vi "Generate Service Config JSON.vi"(0 "service descriptor":T3, 5 "provided interfaces":string[](array[string]), 7 "path":string, 11 "error in":errorcluster) -> (4 "service config JSON":string, 15 "error out":errorcluster)   [LabVIEW 2021, in "NI Measurement Plug-In SDK.lvlib"]
uses:
  NI Measurement Plug-In SDK.lvlib
  TypeDefs/Measurement Details.ctl
  TypeDefs/Measurement Annotation.ctl
  867c5996-9fc4-446f-bc7e-cd1af3184270.vi
  3e130467-15fc-4370-9f76-fa76b7d976c8.vi
  a066e80c-61f1-4c64-8e78-6e3d97fd6b7b.vi
  2858ca83-f95f-4d85-8bb1-5ba8a53c7693.vi
  26abaa1b-7193-4077-a3e4-3b2bfa2f984b.vi
  b2866af8-bc70-4c0d-b595-9f5224cfa858.vi
  0c37daab-07df-4eb5-bca5-1a967d50c5e0.vi
  867c5996-9fc4-446f-bc7e-cd1af3184270.vi/49d2641b-58d2-418d-86ef-5c98235809e6.vi
  867c5996-9fc4-446f-bc7e-cd1af3184270.vi/729eb87d-9ab4-481c-bd0a-7090d6acb718.vi
  3e130467-15fc-4370-9f76-fa76b7d976c8.vi/49d2641b-58d2-418d-86ef-5c98235809e6.vi
  3e130467-15fc-4370-9f76-fa76b7d976c8.vi/729eb87d-9ab4-481c-bd0a-7090d6acb718.vi
  a066e80c-61f1-4c64-8e78-6e3d97fd6b7b.vi/49d2641b-58d2-418d-86ef-5c98235809e6.vi
  a066e80c-61f1-4c64-8e78-6e3d97fd6b7b.vi/729eb87d-9ab4-481c-bd0a-7090d6acb718.vi
  2858ca83-f95f-4d85-8bb1-5ba8a53c7693.vi/49d2641b-58d2-418d-86ef-5c98235809e6.vi
  2858ca83-f95f-4d85-8bb1-5ba8a53c7693.vi/729eb87d-9ab4-481c-bd0a-7090d6acb718.vi
  26abaa1b-7193-4077-a3e4-3b2bfa2f984b.vi/49d2641b-58d2-418d-86ef-5c98235809e6.vi
  26abaa1b-7193-4077-a3e4-3b2bfa2f984b.vi/729eb87d-9ab4-481c-bd0a-7090d6acb718.vi
  b2866af8-bc70-4c0d-b595-9f5224cfa858.vi/49d2641b-58d2-418d-86ef-5c98235809e6.vi
  b2866af8-bc70-4c0d-b595-9f5224cfa858.vi/729eb87d-9ab4-481c-bd0a-7090d6acb718.vi
  0c37daab-07df-4eb5-bca5-1a967d50c5e0.vi/49d2641b-58d2-418d-86ef-5c98235809e6.vi
  0c37daab-07df-4eb5-bca5-1a967d50c5e0.vi/729eb87d-9ab4-481c-bd0a-7090d6acb718.vi
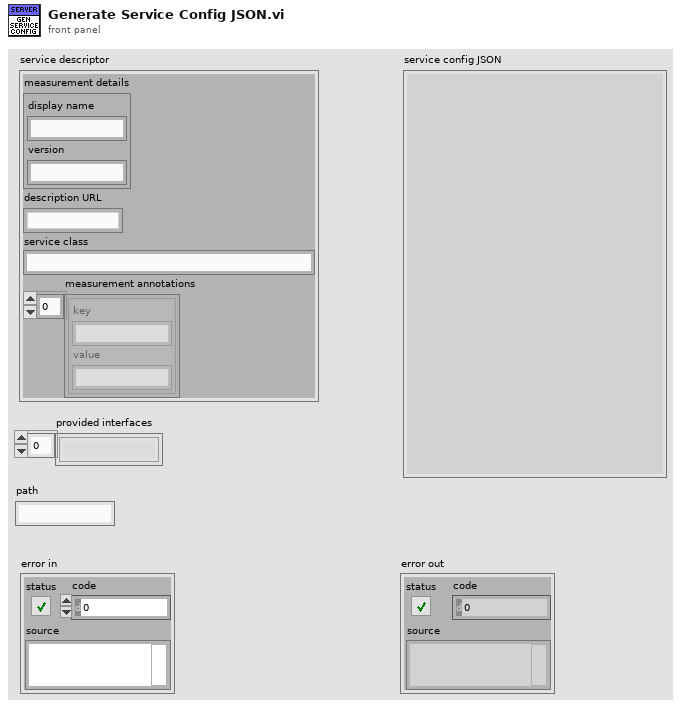
[diagram p1: front panel]
types:
  T1 = typedef "NI Measurement Plug-In SDK.lvlib/Measurement Details.ctl" = cluster{"display name":string, "version":string}
  T2 = typedef "NI Measurement Plug-In SDK.lvlib/Measurement Annotation.ctl" = cluster{"key":string, "value":string}
  T3 = cluster{"measurement details":T1, "description URL":string, "service class":string, "measurement annotations":T2[]}
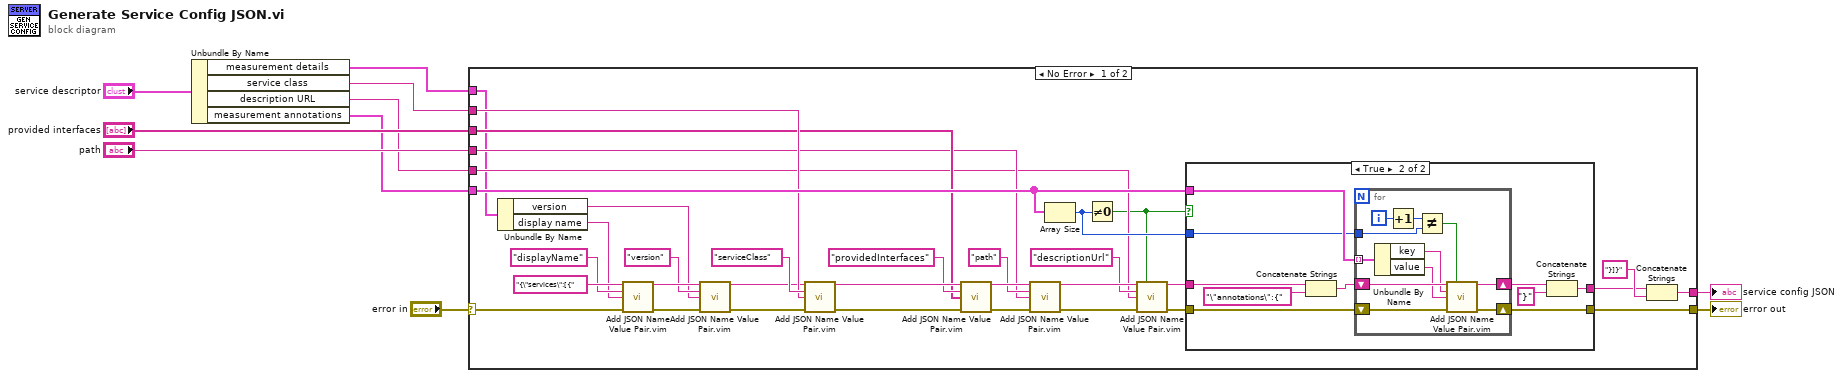
[diagram p0: block diagram]
diagram:
  n1 = Unbundle By Name("service descriptor") -> ("measurement details"=w4:T1, "service class"=w3:string, "description URL"=w2:string, "measurement annotations"=w1:T2[])
  n2 = case shown="No Error" "error in" {
    selector: "error in" -> [w38 w68]
    tunnel: [w42 w68] -> w9
    tunnel: w4 -> [w16 _]
    tunnel: w3 -> [w34 _]
    tunnel: "provided interfaces" -> [w30 _]
    tunnel: [w43 _] -> w7
    tunnel: "path" -> [w26 _]
    tunnel: w2 -> [w21 _]
    tunnel: w1 -> [w41 _]
    frame No Error {
      n3 = Unbundle By Name(w16) -> ("version"=w12:string, "display name"=w15:string)
      n4 = call "Add JSON Name Value Pair.vim"("JSON string in"="{\"services\":[{", "name"="displayName", "value"=w15, "error in"=w38) -> ("JSON string out"=w14:string, "error out"=w18:errorcluster)  [unwired: 10 in]
      n5 = call "Add JSON Name Value Pair.vim"("JSON string in"=w14, "name"="version", "value"=w12, "error in"=w18) -> ("JSON string out"=w11:string, "error out"=w17:errorcluster)  [unwired: 10 in]
      n6 = call "Add JSON Name Value Pair.vim"("JSON string in"=w11, "name"="serviceClass", "value"=w34, "error in"=w17) -> ("JSON string out"=w32:string, "error out"=w33:errorcluster)  [unwired: 10 in]
      n7 = call "Add JSON Name Value Pair.vim"("JSON string in"=w32, "name"="providedInterfaces", "value"=w30, "error in"=w33) -> ("JSON string out"=w28:string, "error out"=w29:errorcluster)  [unwired: 10 in]
      n8 = call "Add JSON Name Value Pair.vim"("JSON string in"=w28, "name"="path", "value"=w26, "error in"=w29) -> ("JSON string out"=w23:string, "error out"=w25:errorcluster)  [unwired: 10 in]
      n9 = Array Size(array=w41) -> (size(s)=w40:i32)
      n10 = Not Equal To 0?(x=w40) -> (x != 0?=w20:bool)
      n11 = call "Add JSON Name Value Pair.vim"("JSON string in"=w23, "include trailing comma"=w20, "name"="descriptionUrl", "value"=w21, "error in"=w25) -> ("JSON string out"=w19:string, "error out"=w24:errorcluster)  [unwired: 9 in]
      n12 = case shown="True" w20 {
        tunnel: w24 -> [w46 w56]
        tunnel: [w46 w55] -> w42
        tunnel: w41 -> [_ w54]
        tunnel: w40 -> [_ w51]
        tunnel: [w45 w48] -> w39
        tunnel: w19 -> [w45 w47]
        frame False {
        }
        frame True {
          n13 = Concatenate Strings(w47, "\"annotations\":{") -> (w52:string)
          n14 = for {
            shift-right: [w62] -> w55
            shift-left: w56 -> [w63]
            tunnel: w54 -> [w65] mode=indexing
            shift-right: [w60] -> w50
            shift-left: w52 -> [w61]
            tunnel: w51 -> [w64]
            i -> [w67]
            n15 = Unbundle By Name(w65) -> ("key"=w57:string, "value"=w58:string)
            n16 = Increment(x=w67) -> (x+1=w66:i32)
            n17 = Not Equal?(x=w66, y=w64) -> (x != y?=w59:bool)
            n18 = call "Add JSON Name Value Pair.vim"("JSON string in"=w61, "include trailing comma"=w59, "name"=w57, "value"=w58, "error in"=w63) -> ("JSON string out"=w60:string, "error out"=w62:errorcluster)  [unwired: 9 in]
          }
          n19 = Concatenate Strings(w50, "}") -> (w48:string)
        }
      }
      n20 = Concatenate Strings(w39, "}]}") -> (w43:string)
    }
    frame Error {
    }
  }
  "error out" <- w9
  "service config JSON" <- w7
